vi "remapWinch.vi"(8 "Reverse Winch Direction?":bool, 9 "Upper Winch Percent":dbl, 10 "Input Percent":dbl, 11 "Lower Winch Percent":dbl) -> (2 "Modified winch duty":dbl)   [LabVIEW 2013]
panel:
  in  "min winch duty (usec)":dbl
  in  "max winch duty (usec)":dbl
  # "All of the below values are determined by the user in the main vi"
  # "TODO: Fill these out for the servo that we're using!"
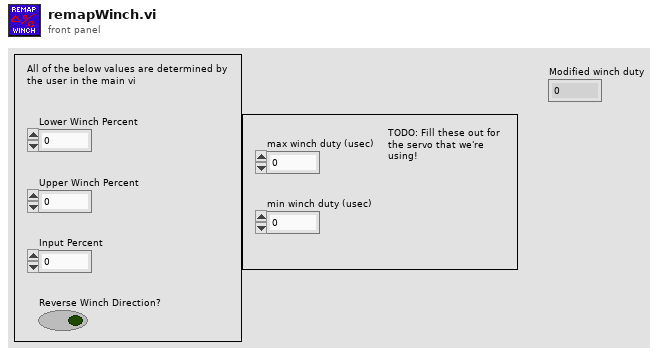
[diagram p1: front panel]
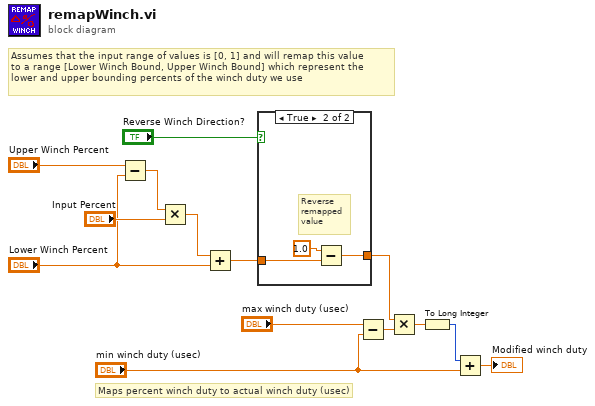
[diagram p0: block diagram]
diagram:
  # "Maps percent winch duty to actual winch duty (usec)"
  # "Assumes that the input range of values is [0, 1] and will remap this value \nto a range [Lower Winch Bound, Upper Winch Bound] which represent the lower and upper bounding percents of the winch duty we use"
  n1 = Subtract(x="Upper Winch Percent", y="Lower Winch Percent") -> (x-y=w13:dbl)
  n2 = Multiply(x=w13, y="Input Percent") -> (x*y=w11:dbl)
  n3 = Add(x=w11, y="Lower Winch Percent") -> (x+y=w7:dbl)
  n4 = case shown="True" "Reverse Winch Direction?" {
    tunnel: w7 -> [w15 w18]
    tunnel: [w15 w16] -> w5
    frame False {
      # "Remapped\nvalue"
    }
    frame True {
      # "Reverse \nremapped\nvalue"
      n5 = Subtract(x=1.0, y=w18) -> (x-y=w16:dbl)
    }
  }
  n6 = Subtract(x="max winch duty (usec)", y="min winch duty (usec)") -> (x-y=w8:dbl)
  n7 = Multiply(x=w5, y=w8) -> (x*y=w4:dbl)
  n8 = To Long Integer(number=w4) -> (32bit integer=w3:i32)
  n9 = Add(x=w3, y="min winch duty (usec)") -> (x+y=→"Modified winch duty":dbl)
